vi "Close All Connections.vi"(7 "Name":string, 8 "error in":errorcluster, 11 "TCP Refs":T1) -> (0 "error out":errorcluster)   [LabVIEW 2013, in "Control Addon Engine.lvlib" / "Network Common API.lvlib"]
uses:
  Network Common API.lvlib
  TCP Refs.ctl
  Network Comm Global Ref.ctl
  <userlib>/STM/Connection Manager/TCP/stm_TCPConnectionMethod.ctl
  <vilib>/NI Veristand/Custom Device Tools/Custom Device Utility Library/Custom Device Utility Library.lvlib
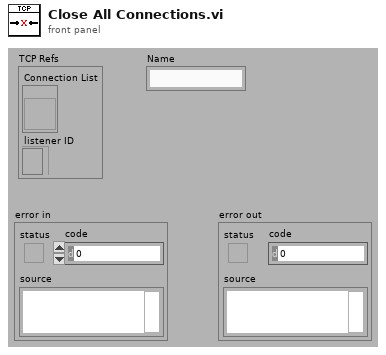
[diagram p1: front panel]
types:
  T1 = typedef "Control Addon Engine.lvlib/Network Common API.lvlib/TCP Refs.ctl" = cluster{"Connection List":T2, "listener ID":refnum<k5>}
  T2 = typedef "Control Addon Engine.lvlib/Network Common API.lvlib/Network Comm Global Ref.ctl" = refnum<vi>
  T3 = typedef "stm_TCPConnectionMethod.ctl" = enum16{"Initialize", "Add Connection", "Set Properties", "Get Connection(s)", "Remove Connection", "Remove All Connections", "Get Connection Count"}
  T4 = typedef "stm_TCP Connection Info.ctl" = cluster{"connection ID":refnum<k5>, "Meta data":T5[]}
  T5 = typedef "stm_MetaDataElement.ctl" = string
  T6 = typedef "stm_TCPConnectionProperties.ctl" = cluster{"Name":string, "Address":string, "Custom":string}
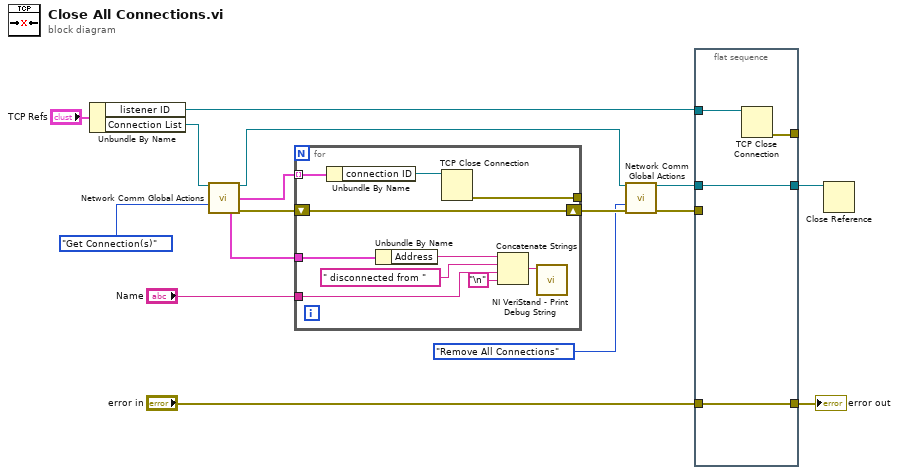
[diagram p0: block diagram]
diagram:
  n1 = Unbundle By Name("TCP Refs") -> ("listener ID"=w1:refnum<k5>, "Connection List"=w2:T2)
  n2 = call "Network Comm Global Actions.vi"("ref in"=w2, "Method"=stm_TCPConnectionMethod."Get Connection(s)") -> ("ref out"=w6:T2, "All Connections"=w13:T4[], "Properties Out"=w4:T6, "error out"=w12:errorcluster)  [unwired: 7 in, 3 out]
  n3 = for {
    tunnel: w13 -> [w18] mode=indexing
    shift-right: [w24] -> w11
    shift-left: w12 -> [w24]
    tunnel: [w25] -> _
    tunnel: "Name" -> [w20]
    tunnel: w4 -> [w19]
    n4 = Unbundle By Name(w18) -> ("connection ID"=w26:refnum<k5>)
    n5 = Unbundle By Name(w19) -> ("Address"=w21:string)
    n6 = TCP Close Connection(connection ID=w26) -> (error out=w25:errorcluster)  [unwired: 2 in, 1 out]
    n7 = Concatenate Strings(w21, " disconnected from " ("string"), w20, "\n") -> (w23:string)
    n8 = call <vilib>:"NI VeriStand - Print Debug String.vi"("Message"=w23) -> ()  [unwired: 10 in, 1 out]
  }
  n9 = call "Network Comm Global Actions.vi"("ref in"=w6, "Method"=stm_TCPConnectionMethod."Remove All Connections", "error in (no error)"=w11) -> ("ref out"=w8:T2, "error out"=w10:errorcluster)  [unwired: 6 in, 5 out]
  n10 = flat-sequence {
    tunnel: w1 -> [w30]
    tunnel: [w29] -> w16
    tunnel: w10 -> [_]
    tunnel: "error in" -> [w29]
    tunnel: [w28] -> _
    tunnel: w8 -> [w27]
    tunnel: [w27] -> w7
    frame #0 {
      n11 = TCP Close Connection(connection ID=w30) -> (error out=w28:errorcluster)  [unwired: 2 in, 1 out]
    }
  }
  n12 = Close Reference(reference=w7) -> ()  [unwired: 1 in, 1 out]
  "error out" <- w16
